vi "DHD1dll.vi"(8 "error in (no error)":errorcluster, 11 "Inputs":cluster{"t":dbl, "D":dbl, "z":dbl[]}) -> (0 "error out":errorcluster, 3 "Outputs":T1)   [LabVIEW 2016]
doc: "subroutine DHD1dll(t, d, z, dhdt_d, dhdt_p, dhdd_t, dhdd_p, dhdp_t, dhdp_d)\n\nCompute partial derivatives of enthalpy w.r.t. T, P, or D at constant T, P, or D as a function of temperature,\ndensity, and composition. See warning in suroutines THERM or ALLPROPS.\n\nINPUTS:\nt -- Temperature [K]\nD -- Molar density [mol/L]\nz -- Composition (array of mole fractions)\n\nOUTPUTS:\ndhdt_d -- dH/dT at constant density [J/(mol-K)]\ndhdt_p -- dH/dT at constant pressure [J/(mol-K)]\ndhdd_t -- dH/drho at constant temperature [(J/mol)/(mol/L)]\ndhdd_p -- dH/drho at constant pressure [(J/mol)/(mol/L)]\ndhdp_t -- dH/dP at constant temperature [J/(mol-kPa)]\ndhdp_d -- dH/dP at constant density [J/(mol-kPa)]"
uses:
  REFPROP.DLL
panel:
  # "REFPROP-DHD1dll.vi"
  # "void  DHD1dll(double *t, double *D, double *z, double *dhdt_d, double *dhdt_p, double *dhdd_t, double *dhdd_p, double *dhdp_t, double *dhdp_d)"
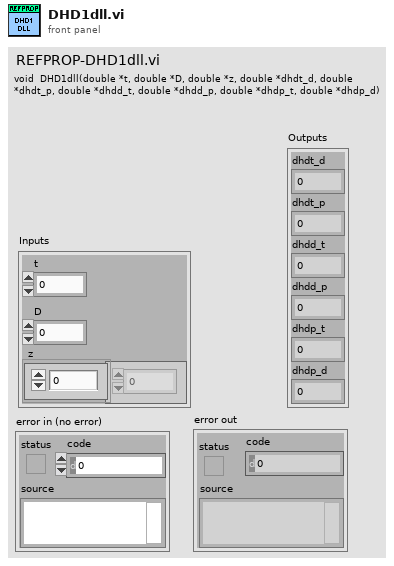
[diagram p1: front panel]
types:
  T1 = cluster{"dhdt_d":dbl, "dhdt_p":dbl, "dhdd_t":dbl, "dhdd_p":dbl, "dhdp_t":dbl, "dhdp_d":dbl}
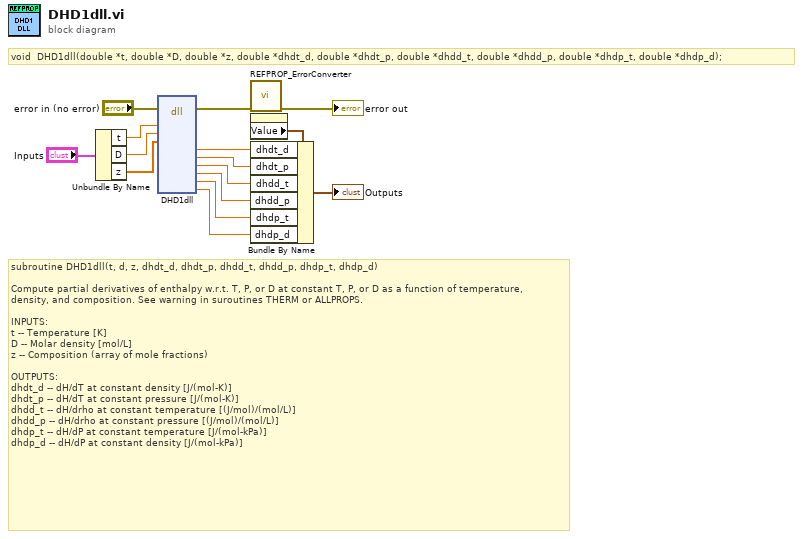
[diagram p0: block diagram]
diagram:
  # "void  DHD1dll(double *t, double *D, double *z, double *dhdt_d, double *dhdt_p, double *dhdd_t, double *dhdd_p, double *dhdp_t, double *dhdp_d);"
  # "subroutine DHD1dll(t, d, z, dhdt_d, dhdt_p, dhdd_t, dhdd_p, dhdp_t, dhdp_d)\n\nCompute partial derivatives of enthalpy w.r.t. T, P, or D at constant T, P, or D as a function of temperature,\ndensity, and composition. See warning in suroutines THERM or ALLPROPS.\n\nINPUTS:\nt -- Temperature [K]\nD -- Molar density [mol/L]\nz -- Composition (array of mole fractions)\n\nOUTPUTS:\ndhdt_d -- dH/dT at constant density [J/(mol-K)]\ndhdt_p -- dH/dT at constant pressure [J/(mol-K)]\ndhdd_t -- dH/drho at constant temperature [(J/mol)/(mol/L)]\ndhdd_p -- dH/drho at constant pressure [(J/mol)/(mol/L)]\ndhdp_t -- dH/dP at constant temperature [J/(mol-kPa)]\ndhdp_d -- dH/dP at constant density [J/(mol-kPa)]"
  n1 = Unbundle By Name("Inputs") -> ("t"=w9:dbl, "D"=w10:dbl, "z"=w11:dbl[])
  n2 = dll-call lib="S:/009 - Testing/02 - Performance Testing/REFPROP/REFPROP.*" fn="DHD1dll"(error in="error in (no error)", "t"=w9, "D"=w10, "z"=w11) -> (error out=w15:errorcluster, "dhdt_d"=w1:dbl, "dhdt_p"=w6:dbl, "dhdd_t"=w5:dbl, "dhdd_p"=w4:dbl, "dhdp_t"=w3:dbl, "dhdp_d"=w2:dbl)  [unwired: 12 in, 1 out]
  n3 = call "REFPROP_ErrorConverter.vi"("error in (no error)"=w15) -> ("error out"=→"error out":errorcluster)  [unwired: 10 in]
  n4 = property on="Outputs" class="Clust (strict)"() -> ("Value"=w7:T1)  [unwired: 2 in, 2 out]
  n5 = Bundle By Name(cluster=w7, "dhdt_d"=w1, "dhdt_p"=w6, "dhdd_t"=w5, "dhdd_p"=w4, "dhdp_t"=w3, "dhdp_d"=w2) -> (→"Outputs":T1)
